vi "SGInitParametersdefault.vi"(11 "Refnum in":refnum<k21>) -> (3 "Refnum out":refnum<k21>)   [LabVIEW 2013, in "IRIO.lvlib"]
uses:
  IRIO.lvlib
  <vilib>/rvi/DataTransferAndStorage/Container/Common/niFpgaContainerExecOnDevCompGetState.vi
  <vilib>/rvi/DataTransferAndStorage/Register/Emulation/niFpgaRegisterEmulationFpgaImpl.vi
  <instcachedir>/0/niFpgaRegisterEmulationFpgaImpl_DCF4BC0110594B98B44A971D60CEEC4D.lvgen/niFpgaRegisterEmulationFpgaImpl_DCF4BC0110594B98B44A971D60CEEC4D_009.vi
  <vilib>/rvi/DataTransferAndStorage/Container/Common/niFpgaContainerGetUniqueNameForEmu.vi
  <vilib>/rvi/DataTransferAndStorage/Container/XNode/niFpgaContainer.xnode
  <vilib>/rvi/DataTransferAndStorage/Register/Emulation/niFpgaRegisterEmulationRefIn.vi
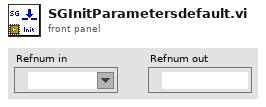
[diagram p1: front panel]
types:
  T1 = cluster{"AOEnable":bool, "AO0":i32, "SGUpdateRate":u32, "SGPhase":u32, "SGFreq":u32, "SGAmp":u16, "SGSignalType":u8, "SimulatedAO":i32}
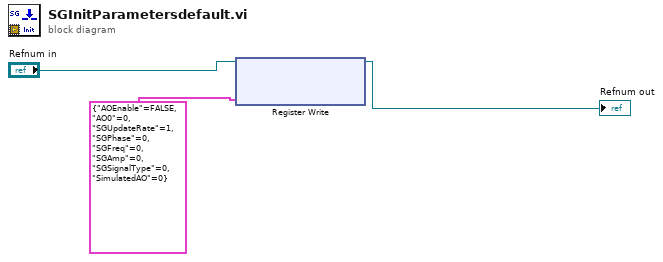
[diagram p0: block diagram]
diagram:
  n1 = xnode "Register Write"("Data"=T1 {"AOEnable"=FALSE, "AO0"=0, "SGUpdateRate"=1, "SGPhase"=0, "SGFreq"=0, "SGAmp"=0, "SGSignalType"=0, "SimulatedAO"=0} ("Cluster"), "Register In"="Refnum in") -> ("Register Out"=→"Refnum out":refnum<k21>)
